vi "VI Tree.vi"   [LabVIEW 2015, in "Fluke 28x Series.lvlib"]
doc: "This is the instrument driver for the Fluke 28x. The VI Tree displays all the user-callable VIs of the instrument driver in an organized table."
uses:
  <instrlib>/Fluke 28x Series/Fluke 28x Series.lvlib
panel:
  # "(c) 2009-2014 National Instruments.  ALL RIGHTS RESERVED."
  # "SEE DIAGRAM\nFOR VI TREE."
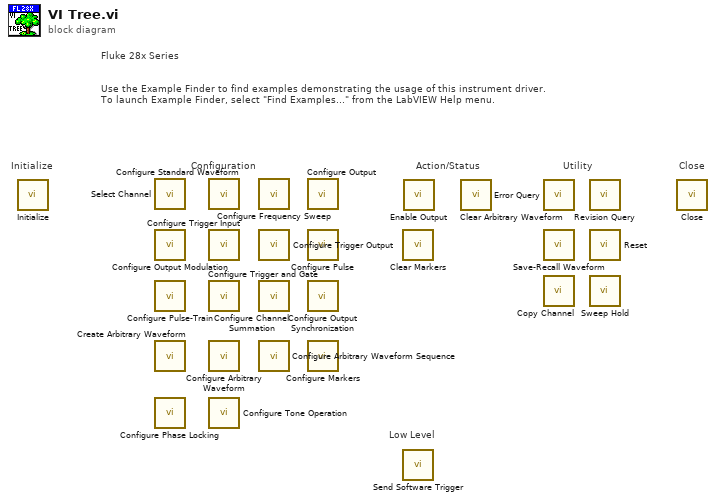
[diagram p0: block diagram]
diagram:
  # "Low Level"
  # "Fluke 28x Series\n\n\nUse the Example Finder to find examples demonstrating the usage of this instrument driver.\nTo launch Example Finder, select \"Find Examples...\" from the LabVIEW Help menu."
  # "Configuration"
  # "Utility"
  # "Action/Status"
  # "Close"
  # "Initialize"
  n1 = call <instrlib>:"Initialize.vi"() -> ()  [unwired: 10 in, 2 out]
  n2 = call <instrlib>:"Select Channel.vi"() -> ()  [unwired: 10 in, 2 out]
  n3 = call <instrlib>:"Configure Output Modulation.vi"() -> ()  [unwired: 10 in, 2 out]
  n4 = call <instrlib>:"Configure Pulse-Train.vi"() -> ()  [unwired: 10 in, 2 out]
  n5 = call <instrlib>:"Create Arbitrary Waveform.vi"() -> ()  [unwired: 10 in, 2 out]
  n6 = call <instrlib>:"Configure Phase Locking.vi"() -> ()  [unwired: 10 in, 2 out]
  n7 = call <instrlib>:"Configure Standard Waveform.vi"() -> ()  [unwired: 10 in, 2 out]
  n8 = call <instrlib>:"Configure Trigger Input.vi"() -> ()  [unwired: 10 in, 2 out]
  n9 = call <instrlib>:"Configure Trigger and Gate.vi"() -> ()  [unwired: 10 in, 2 out]
  n10 = call <instrlib>:"Configure Arbitrary Waveform.vi"() -> ()  [unwired: 18 in, 2 out]
  n11 = call <instrlib>:"Configure Tone Operation.vi"() -> ()  [unwired: 10 in, 2 out]
  n12 = call <instrlib>:"Configure Frequency Sweep.vi"() -> ()  [unwired: 14 in, 2 out]
  n13 = call <instrlib>:"Configure Trigger Output.vi"() -> ()  [unwired: 10 in, 2 out]
  n14 = call <instrlib>:"Configure Channel Summation.vi"() -> ()  [unwired: 10 in, 2 out]
  n15 = call <instrlib>:"Configure Arbitrary Waveform Sequence.vi"() -> ()  [unwired: 10 in, 2 out]
  n16 = call <instrlib>:"Configure Output.vi"() -> ()  [unwired: 10 in, 2 out]
  n17 = call <instrlib>:"Configure Pulse.vi"() -> ()  [unwired: 10 in, 2 out]
  n18 = call <instrlib>:"Configure Output Synchronization.vi"() -> ()  [unwired: 10 in, 2 out]
  n19 = call <instrlib>:"Configure Markers.vi"() -> ()  [unwired: 10 in, 2 out]
  n20 = call <instrlib>:"Clear Markers.vi"() -> ()  [unwired: 10 in, 2 out]
  n21 = call <instrlib>:"Send Software Trigger.vi"() -> ()  [unwired: 10 in, 2 out]
  n22 = call <instrlib>:"Enable Output.vi"() -> ()  [unwired: 10 in, 2 out]
  n23 = call <instrlib>:"Clear Arbitrary Waveform.vi"() -> ()  [unwired: 10 in, 2 out]
  n24 = call <instrlib>:"Error Query.vi"() -> ()  [unwired: 8 in, 4 out]
  n25 = call <instrlib>:"Save-Recall Waveform.vi"() -> ()  [unwired: 10 in, 2 out]
  n26 = call <instrlib>:"Copy Channel.vi"() -> ()  [unwired: 10 in, 2 out]
  n27 = call <instrlib>:"Revision Query.vi"() -> ()  [unwired: 8 in, 4 out]
  n28 = call <instrlib>:"Reset.vi"() -> ()  [unwired: 10 in, 2 out]
  n29 = call <instrlib>:"Sweep Hold.vi"() -> ()  [unwired: 10 in, 2 out]
  n30 = call <instrlib>:"Close.vi"() -> ()  [unwired: 11 in, 1 out]
